vi "gun_speed_feed_forward.vi"(11 "RPM":dbl) -> (3 "Power":dbl)   [LabVIEW 2011]
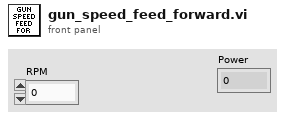
[diagram p1: front panel]
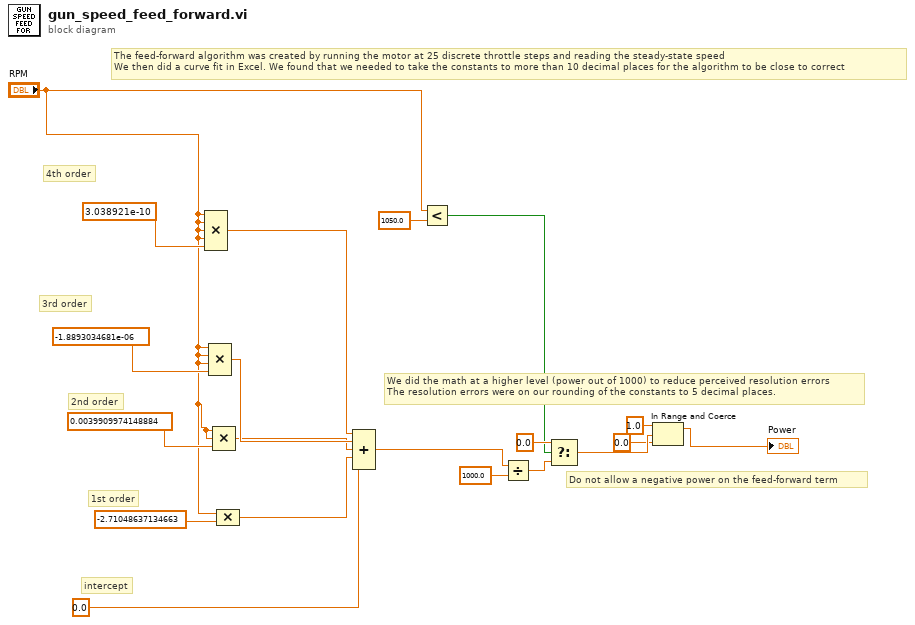
[diagram p0: block diagram]
diagram:
  # "Do not allow a negative power on the feed-forward term"
  # "We did the math at a higher level (power out of 1000) to reduce perceived resolution errors\nThe resolution errors were on our rounding of the constants to 5 decimal places."
  # "The feed-forward algorithm was created by running the motor at 25 discrete throttle steps and reading the steady-state speed\nWe then did a curve fit in Excel. We found that we needed to take the constants to more than 10 decimal places for the algorithm to be close to correct"
  # "intercept"
  # "1st order"
  # "2nd order"
  # "3rd order"
  # "4th order"
  n1 = Compound Arithmetic op=MULTIPLY("RPM", "RPM", "RPM", "RPM", 3.038921e-10) -> (w16:dbl)
  n2 = Compound Arithmetic op=MULTIPLY("RPM", "RPM", "RPM", -1.8893034681e-06) -> (w15:dbl)
  n3 = Compound Arithmetic op=MULTIPLY("RPM", "RPM", 0.0039909974148884) -> (w14:dbl)
  n4 = Compound Arithmetic op=MULTIPLY("RPM", -2.71048637134663) -> (w13:dbl)
  n5 = Compound Arithmetic op=ADD(w16, w15, w14, w13, 0.0) -> (w11:dbl)
  n6 = Less?(x="RPM", y=1050.0) -> (x < y?=w5:bool)
  n7 = Divide(x=w11, y=1000.0) -> (x/y=w9:dbl)
  n8 = Select(t=0.0, s=w5, f=w9) -> (s? t:f=w4:dbl)
  n9 = In Range and Coerce(upper limit=1.0, x=w4, lower limit=0.0) -> (coerced(x)=→"Power":dbl)  [unwired: 1 out]
